vi "LH_GetListLength.vi"(3 "InputList":refnum<class "ListHead.lvclass">) -> (0 "NodeNum":u32, 1 "OutputList":refnum<class "ListHead.lvclass">)   [LabVIEW 2014, in "ListHead.lvclass"]
uses:
  ListHead.lvclass
  ListHead.lvclass/ListHead.ctl
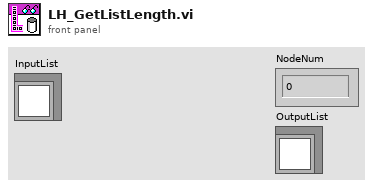
[diagram p1: front panel]
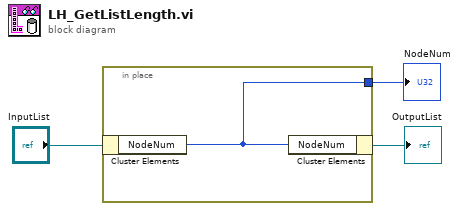
[diagram p0: block diagram]
diagram:
  n1 = in-place {
    in-place-border: [w4] -> w2
    n2 = in-place-cluster #1("InputList") -> ("NodeNum"=w4:u32)
    n3 = in-place-cluster #1("NodeNum"=w4) -> (→"OutputList":refnum<class "ListHead.lvclass">)
  }
  "NodeNum" <- w2
